vi "Configure CAN.vi"(8 "error in":errorcluster, 11 "HSU MCU V2 Monitor CFG in":refnum<class "HSU MCU V2 CFG.lvclass">) -> (0 "error out":errorcluster, 3 "HSU MCU V2 Monitor CFG out":refnum<class "HSU MCU V2 CFG.lvclass">)   [LabVIEW 2023, in "HSU MCU V2 CFG.lvclass"]
uses:
  HSU MCU V2 CFG.lvclass
  Configurations/CFG JSON/CFG JSON.lvclass
  Protocols/ICAN/ICAN.lvclass
  HSU MCU V2 CFG.lvclass/HSU MCU V2 CFG.ctl
  60c77de9-abfb-4302-865d-68a0323ddca5.vi
  <vilib>/JDP Science/JSONtext/Next JSON Value.vi
  <vilib>/JDP Science/JSONtext/String Subset.vi
  60c77de9-abfb-4302-865d-68a0323ddca5.vi/a4169a97-72fc-4003-a778-603cf20cafa0.vi
  <vilib>/JDP Science/JSONtext/Parsing/Advance past next JSON Value (inlined COPY).vi
  <vilib>/JDP Science/JSONtext/Parsing/Advance past whitespace.vi
  <vilib>/JDP Science/JSONtext/Parsing/Advance past String.vi
  <vilib>/JDP Science/JSONtext/Parsing/Advance past Number.vi
  <vilib>/JDP Science/JSONtext/Parsing/Advance past Line Ending.vi
  <vilib>/JDP Science/JSONtext/Parsing/Parse Full Path or Item Name.vi
  <vilib>/JDP Science/JSONtext/Parsing/Advance past Array.vi
  <vilib>/JDP Science/JSONtext/Parsing/Advance past Object.vi
  <vilib>/JDP Science/JSONtext/support/Error Cluster From Code.vi
  <vilib>/JDP Science/JSONtext/Offset/Find Item Locations by Path.vi
  <vilib>/JDP Science/JSONtext/JSON text to Variant.vi
  <vilib>/Utility/error.llb/Error Cluster From Error Code.vi
  <vilib>/JDP Science/JSONtext/LVClass Serializer/JSONtext LVClass Serializer.lvclass
  <vilib>/JDP Science/JSONtext/JSONtext.lvlib
  Configurations/CFG Base/CFG Base.lvclass
  D:/git/HAL/HAL/Configurations/CFG JSON/CFG JSON.lvclass
  D:/git/HAL/HAL/Configurations/CFG Base/CFG Base.lvclass
  D:/git/HAL/HAL/Devices/HSU MCU V2 CFG/HSU MCU V2 CFG/HSU MCU V2 CFG.lvclass
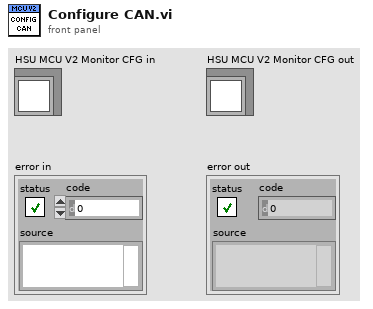
[diagram p1: front panel]
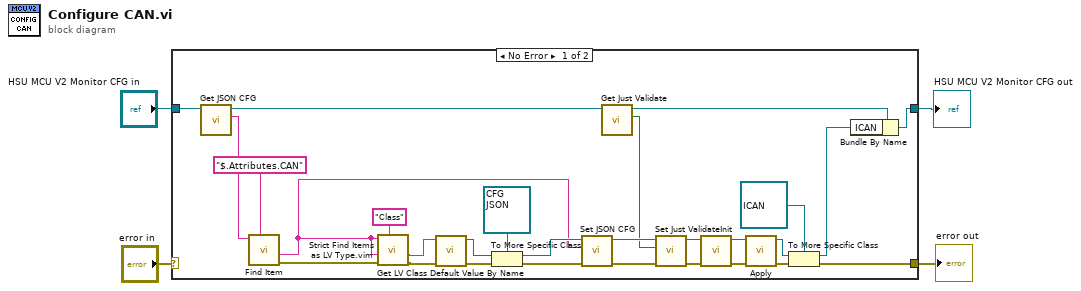
[diagram p0: block diagram]
diagram:
  n1 = case shown="No Error" "error in" {
    selector: "error in" -> [_ w32]
    tunnel: [w23 w32] -> w3
    tunnel: [w6 w31] -> w1
    tunnel: "HSU MCU V2 Monitor CFG in" -> [w30 w31]
    frame No Error {
      n2 = call "Get JSON CFG.vi"("CFG JSON in"=w30) -> ("<JSON> CFG"=w16:string, "CFG JSON out"=w9:refnum<class "HSU MCU V2 CFG.lvclass">)  [unwired: 9 in]
      n3 = call <vilib>:"Find Item.vi"("$Path or Item Name"="$.Attributes.CAN", "JSON"=w16) -> ("error out"=w15:errorcluster, "<JSON>"=w14:string)  [unwired: 6 in, 2 out]
      n4 = call "Strict Find Items as LV Type.vim"("$Path or Item Name"="Class", "error in"=w15, "Data Type and Default Value"=w14, "<JSON>"=w14) -> ("error out"=w11:errorcluster, "Data out"=w12:string)  [unwired: 5 in, 1 out]
      n5 = call <vilib>:"Get LV Class Default Value By Name.vi"("error in (no error)"=w11, "class name"=w12) -> ("error out"=w29:errorcluster, "object"=w27:refnum<class>)  [unwired: 8 in]
      n6 = To More Specific Class(target class=refnum<class "CFG JSON.lvclass"> refnum ("ICommunicate.lvclass"), reference=w27, error in=w29) -> (specific class reference=w18:refnum<class "CFG JSON.lvclass">, error out=w10:errorcluster)
      n7 = call "Set JSON CFG.vi"("<JSON> CFG"=w14, "CFG JSON in"=w18) -> ("CFG JSON out"=w19:refnum<class "CFG JSON.lvclass">)  [unwired: 9 in]
      n8 = call "Get Just Validate.vi"("CFG Base in"=w9) -> ("Just Validate"=w7:bool, "CFG Base out"=w5:refnum<class "HSU MCU V2 CFG.lvclass">)  [unwired: 9 in]
      n9 = call "Set Just Validate.vi"("Just Validate"=w7, "CFG Base in"=w19) -> ("CFG Base out"=w8:refnum<class "CFG JSON.lvclass">)  [unwired: 9 in]
      n10 = call-dynamic "Init.vi"("error in"=w10, "CFG Base in"=w8) -> ("error out"=w26:errorcluster, "CFG Base out"=w24:refnum<class "CFG JSON.lvclass">)  [unwired: 8 in]
      n11 = call-dynamic "Apply.vi"("error in"=w26, "CFG Base in"=w24) -> ("error out"=w25:errorcluster, "CFG Base out"=w22:refnum<class "CFG JSON.lvclass">)  [unwired: 8 in]
      n12 = To More Specific Class(target class=refnum<class "ICAN.lvclass"> refnum ("ICAN.lvclass"), reference=w22, error in=w25) -> (specific class reference=w20:refnum<class "ICAN.lvclass">, error out=w23:errorcluster)
      n13 = Bundle By Name(cluster=w5, "ICAN"=w20) -> (w6:refnum<class "HSU MCU V2 CFG.lvclass">)
    }
    frame Error {
    }
  }
  "error out" <- w3
  "HSU MCU V2 Monitor CFG out" <- w1
